vi "Read DC Pins.vi"(8 "error in (no error)":errorcluster, 11 "DCLeakage in":refnum<class "DCLeakage.lvclass">) -> (0 "error out":errorcluster, 2 "DC Pins":string[](array[string]), 3 "DCLeakage out":refnum<class "DCLeakage.lvclass">)   [LabVIEW 2018, in "SeqAuto Evaluations.lvlib" / "DCLeakage.lvclass"]
uses:
  DCLeakage.lvclass
  DCLeakage.lvclass/DCLeakage.ctl
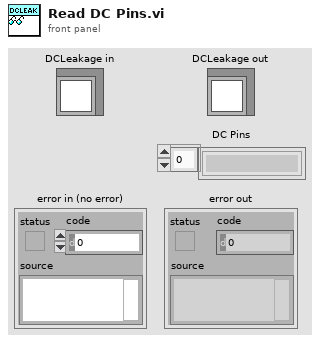
[diagram p1: front panel]
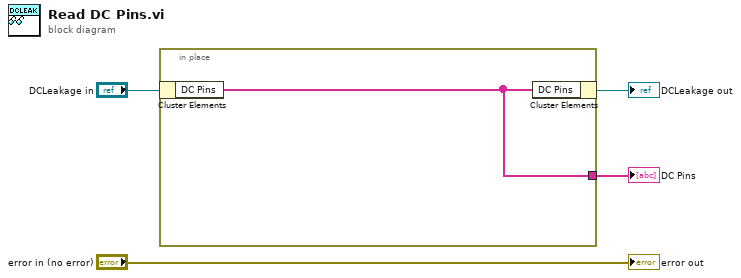
[diagram p0: block diagram]
diagram:
  n1 = in-place {
    in-place-border: [w5] -> w1
    n2 = in-place-cluster #1("DCLeakage in") -> ("DC Pins"=w5:string[])
    n3 = in-place-cluster #1("DC Pins"=w5) -> (→"DCLeakage out":refnum<class "DCLeakage.lvclass">)
  }
  "DC Pins" <- w1
  "error out" <- "error in (no error)"
